vi "Write Values to File.vi"(0 "Image Name":string="20170125_164904.835_IMGA.png", 1 "Right Spindle (microns)":dbl, 3 "Left Spindle (microns)":dbl, 4 "Center Spindle (microns)":dbl, 5 "Center Spindle (Pixels)":dbl, 6 "Error at file writing":errorcluster, 7 "file path (dialog if empty)":path, 8 "Left Spindle (Pixels)":dbl, 9 "Right Spindle (Pixels)":dbl) -> (14 "new file path (Not A Path if cancelled)":path, 19 "Error out at file writing":errorcluster)   [LabVIEW 2016]
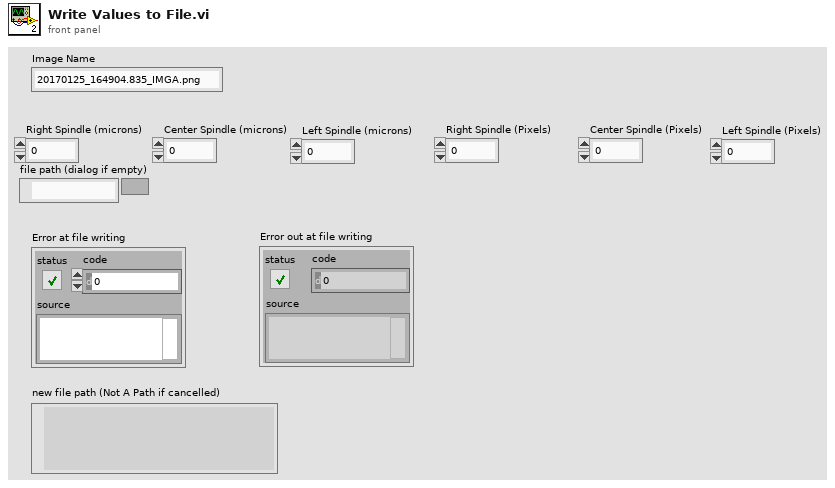
[diagram p1: front panel]
types:
  T1 = enum16{"open", "replace", "create", "open or create", "replace or create", "replace or create with confirmation"}
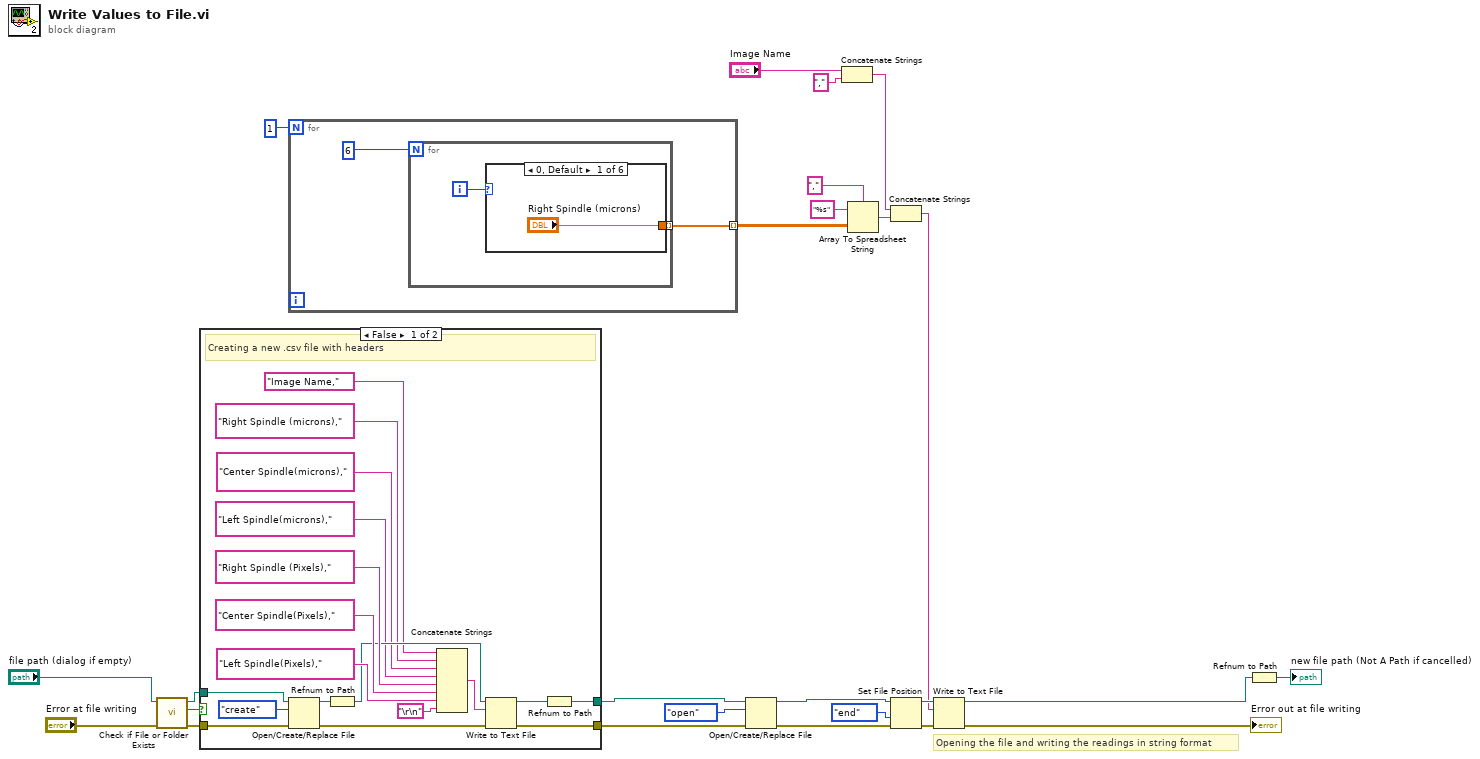
[diagram p0: block diagram]
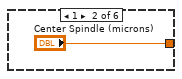
[diagram p3: hidden frame]
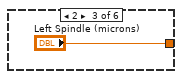
[diagram p4: hidden frame]
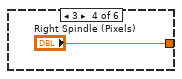
[diagram p5: hidden frame]
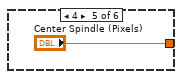
[diagram p6: hidden frame]
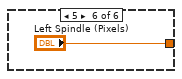
[diagram p7: hidden frame]
diagram:
  # "Opening the file and writing the readings in string format"
  n1 = call <vilib>:"Check if File or Folder Exists.vi"("error in (no error)"="Error at file writing", "path"="file path (dialog if empty)") -> ("error out"=w4:errorcluster, "file or folder exists?"=w5:bool, "dup path"=w2:path)  [unwired: 7 in]
  n2 = case shown="False" w5 {
    tunnel: [w31 w45] -> w3
    tunnel: w4 -> [w41 w45]
    tunnel: w2 -> [w43 w44]
    tunnel: [w33 w44] -> w1
    frame False {
      # "Creating a new .csv file with headers"
      n3 = Open/Create/Replace File(file path (use dialog)=w43, error in=w41, operation (0:open)=T1."create") -> (refnum out=w40:refnum<file>, error out=w32:errorcluster)  [unwired: 3 in, 1 out]
      n4 = Refnum to Path(1:w40) -> (0:w35:path)
      n5 = Concatenate Strings("Image Name," ("string"), "Right Spindle (microns)," ("string"), "Center Spindle(microns)," ("string"), "Left Spindle(microns)," ("string"), "Right Spindle (Pixels)," ("string"), "Center Spindle(Pixels)," ("string"), "Left Spindle(Pixels)," ("string"), "\r\n") -> (w36:string)
      n6 = Write to Text File(file (use dialog)=w35, text=w36, error in=w32) -> (refnum out=w34:refnum<file>, error out=w31:errorcluster)  [unwired: 1 in, 1 out]
      n7 = Refnum to Path(1:w34) -> (0:w33:path)
    }
    frame True {
      # "If the file exists then the data is wriiten to .csv file"
    }
  }
  n8 = for {
    N: 1 -> [_]
    tunnel: [w46] -> w8 mode=indexing
    n9 = for {
      N: 6 ("Numeric") -> [_]
      tunnel: [w48] -> w46 mode=indexing
      i -> [w49]
      n10 = case shown="0, Default" w49 {
        tunnel: ["Right Spindle (microns)" "Center Spindle (microns)" "Left Spindle (microns)" "Right Spindle (Pixels)" "Center Spindle (Pixels)" "Left Spindle (Pixels)"] -> w48
        frame 0, Default {
        }
        frame 1 {
        }
        frame 2 {
        }
        frame 3 {
        }
        frame 4 {
        }
        frame 5 {
        }
      }
    }
  }
  n11 = Open/Create/Replace File(file path (use dialog)=w1, error in=w3, operation (0:open)=T1."open") -> (refnum out=w21:refnum<file>, error out=w12:errorcluster)  [unwired: 3 in, 1 out]
  n12 = Concatenate Strings("Image Name", "," ("delimiter (\\t)")) -> (w17:string)
  n13 = Array To Spreadsheet String(delimiter (Tab)="," ("delimiter (\\t)"), array=w8, 3:"%s" ("format string")) -> (spreadsheet string=w15:string)
  n14 = Concatenate Strings(w17, w15) -> (w20:string)
  n15 = Set File Position(refnum=w21, from (0:start)=enum16{"start", "end", "current"}."end", error in=w12) -> (refnum out=w23:refnum<file>, error out=w19:errorcluster)  [unwired: 1 in]
  n16 = Write to Text File(file (use dialog)=w23, text=w20, error in=w19) -> (refnum out=w10:refnum<file>, error out=→"Error out at file writing":errorcluster)  [unwired: 1 in, 1 out]
  n17 = Refnum to Path(1:w10) -> (0:→"new file path (Not A Path if cancelled)":path)
